vi "Get Data Version.vi"(8 "error in (no error)":errorcluster, 11 "UDPlog Transfer Rx Configuration in":refnum<class "UDPlog Transfer Rx Configuration.lvclass">) -> (0 "error out":errorcluster, 2 "data version":T1, 3 "UDPlog Transfer Rx Configuration out":refnum<class "UDPlog Transfer Rx Configuration.lvclass">)   [LabVIEW 2023, in "UDPlog.lvlib" / "UDPlog Transfer Rx Configuration.lvclass"]
uses:
  UDPlog Transfer Rx Configuration.lvclass
  UDPlog Transfer Rx Configuration.lvclass/UDPlog Transfer Rx Configuration.ctl
  <vilib>/AddOns/VeriStand Custom Device Scripting APIs/Data Sharing Framework/DSF Core.lvlibp/Classes/Configuration/Configuration.lvclass
  <vilib>/AddOns/VeriStand Custom Device Scripting APIs/Data Sharing Framework/DSF Core.lvlibp/Typedefs/DSF Version Info.ctl
  <vilib>/AddOns/VeriStand Custom Device Scripting APIs/Data Sharing Framework/DSF Core.lvlibp
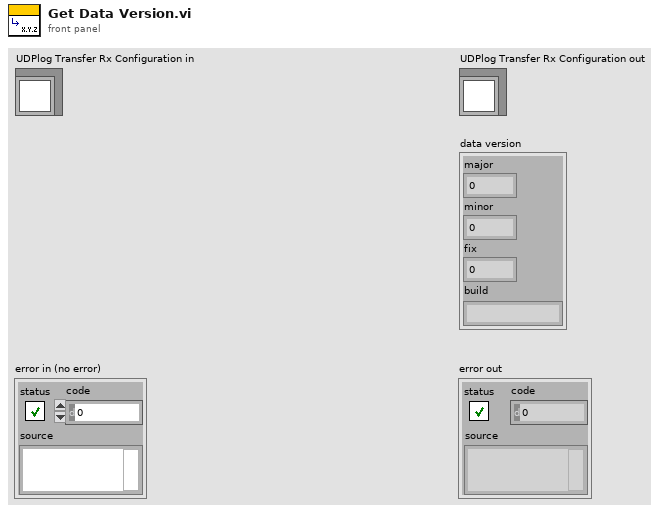
[diagram p1: front panel]
types:
  T1 = typedef "DSF Core.lvlibp/DSF Version Info.ctl" = cluster{"major":u32, "minor":u32, "fix":u32, "build":string}
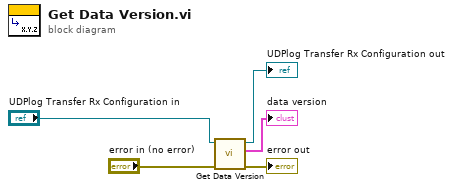
[diagram p0: block diagram]
diagram:
  n1 = call-parent "Get Data Version.vi"("error in (no error)"="error in (no error)", "Configuration in"="UDPlog Transfer Rx Configuration in") -> ("error out"=→"error out":errorcluster, "data version"=→"data version":T1, "Configuration out"=→"UDPlog Transfer Rx Configuration out":refnum<class "UDPlog Transfer Rx Configuration.lvclass">)  [unwired: 7 in]
